vi "OdaNaRadost.vi"(11 "NXT/EV3":T1) -> (3 "NXT/EV3 2":T1)   [LabVIEW 2016]
uses:
  <vilib>/NXT/Subs/LVHSConnector.ctl
  <vilib>/NXT/LegoClasses/BrickReference/BrickReference.lvclass
  <vilib>/NXT/Block Support/NXT_OutputPort.ctl
  <vilib>/NXT/Dual Mode Library/Display/drawText_Center.vi
  <vilib>/NXT/Dual Mode Library/Sound/PlayE.vi
  <vilib>/NXT/Dual Mode Library/Sound/PlayF.vi
  <vilib>/NXT/Dual Mode Library/Sound/PlayG.vi
  <vilib>/NXT/Dual Mode Library/Sound/PlayD.vi
  <vilib>/NXT/Dual Mode Library/Sound/PlayC.vi
  <vilib>/NXT/Dual Mode Library/Waits/Wait_Num.vi
  <vilib>/NXT/NXTIO Xnodes/NXTIONodeSubVIs/NXTMoveMotors.vi
  <vilib>/NXT/NXTIO Xnodes/NXTIONodeSubVIs/NXTStopMotors.vi
  <vilib>/NXT/NXTIO Xnodes/AddressXNode/NXTIOAddress.xnode
  <vilib>/NXT/NXTIO Xnodes/NXTIOXNode/NXTIO.xnode
panel:
  in  "Poèet opakování":i32
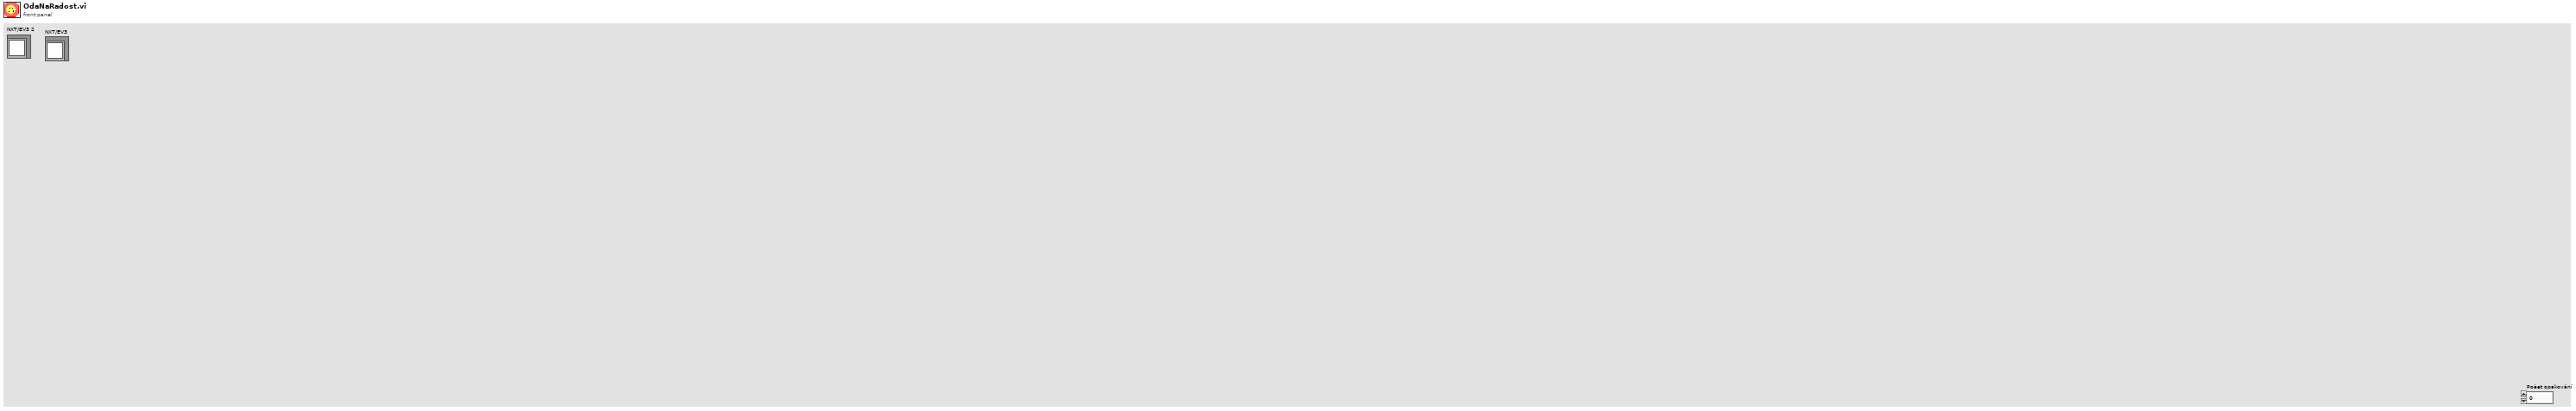
[diagram p1: front panel]
types:
  T1 = typedef "LVHSConnector.ctl" = refnum<class "BrickReference.lvclass">
  T2 = typedef "NXT_OutputPort.ctl" = u8
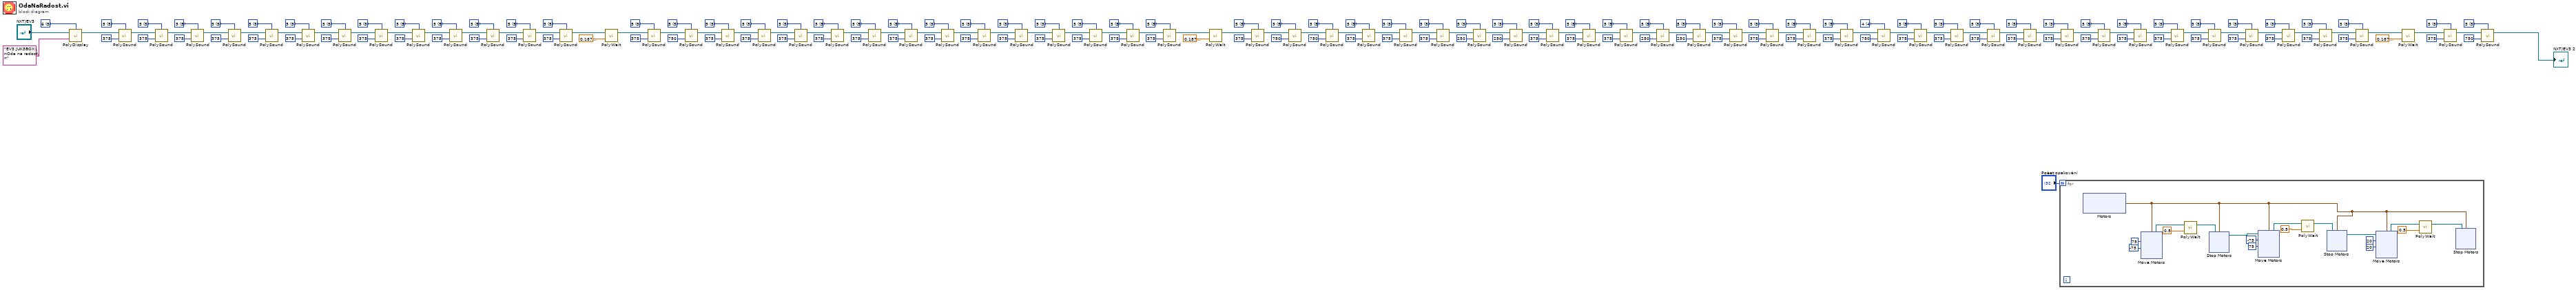
[diagram p0: block diagram]
diagram:
  w47 = u16 5 items=["3"=3, "4"=4, "5"=5, "6"=6, "7"=7] ("Octave")
  w50 = u16 5 items=["3"=3, "4"=4, "5"=5, "6"=6, "7"=7] ("Octave")
  w41 = u16 5 items=["3"=3, "4"=4, "5"=5, "6"=6, "7"=7] ("Octave")
  w36 = u16 5 items=["3"=3, "4"=4, "5"=5, "6"=6, "7"=7] ("Octave")
  w33 = u16 5 items=["3"=3, "4"=4, "5"=5, "6"=6, "7"=7] ("Octave")
  w32 = u16 5 items=["3"=3, "4"=4, "5"=5, "6"=6, "7"=7] ("Octave")
  w29 = u16 5 items=["3"=3, "4"=4, "5"=5, "6"=6, "7"=7] ("Octave")
  w20 = u16 5 items=["3"=3, "4"=4, "5"=5, "6"=6, "7"=7] ("Octave")
  w23 = u16 5 items=["3"=3, "4"=4, "5"=5, "6"=6, "7"=7] ("Octave")
  w24 = u16 5 items=["3"=3, "4"=4, "5"=5, "6"=6, "7"=7] ("Octave")
  w27 = u16 5 items=["3"=3, "4"=4, "5"=5, "6"=6, "7"=7] ("Octave")
  w13 = u16 5 items=["3"=3, "4"=4, "5"=5, "6"=6, "7"=7] ("Octave")
  w10 = u16 5 items=["3"=3, "4"=4, "5"=5, "6"=6, "7"=7] ("Octave")
  w9 = u16 5 items=["3"=3, "4"=4, "5"=5, "6"=6, "7"=7] ("Octave")
  w6 = u16 5 items=["3"=3, "4"=4, "5"=5, "6"=6, "7"=7] ("Octave")
  w53 = u16 4 items=["3"=3, "4"=4, "5"=5, "6"=6, "7"=7] ("Octave")
  w60 = u16 5 items=["3"=3, "4"=4, "5"=5, "6"=6, "7"=7] ("Octave")
  w67 = u16 5 items=["3"=3, "4"=4, "5"=5, "6"=6, "7"=7] ("Octave")
  w70 = u16 5 items=["3"=3, "4"=4, "5"=5, "6"=6, "7"=7] ("Octave")
  w71 = u16 5 items=["3"=3, "4"=4, "5"=5, "6"=6, "7"=7] ("Octave")
  w74 = u16 5 items=["3"=3, "4"=4, "5"=5, "6"=6, "7"=7] ("Octave")
  w57 = u16 5 items=["3"=3, "4"=4, "5"=5, "6"=6, "7"=7] ("Octave")
  w54 = u16 5 items=["3"=3, "4"=4, "5"=5, "6"=6, "7"=7] ("Octave")
  w91 = u16 5 items=["3"=3, "4"=4, "5"=5, "6"=6, "7"=7] ("Octave")
  w94 = u16 5 items=["3"=3, "4"=4, "5"=5, "6"=6, "7"=7] ("Octave")
  w95 = u16 5 items=["3"=3, "4"=4, "5"=5, "6"=6, "7"=7] ("Octave")
  w98 = u16 5 items=["3"=3, "4"=4, "5"=5, "6"=6, "7"=7] ("Octave")
  w84 = u16 5 items=["3"=3, "4"=4, "5"=5, "6"=6, "7"=7] ("Octave")
  w81 = u16 5 items=["3"=3, "4"=4, "5"=5, "6"=6, "7"=7] ("Octave")
  w80 = u16 5 items=["3"=3, "4"=4, "5"=5, "6"=6, "7"=7] ("Octave")
  w77 = u16 5 items=["3"=3, "4"=4, "5"=5, "6"=6, "7"=7] ("Octave")
  w142 = u16 5 items=["3"=3, "4"=4, "5"=5, "6"=6, "7"=7] ("Octave")
  w145 = u16 5 items=["3"=3, "4"=4, "5"=5, "6"=6, "7"=7] ("Octave")
  w136 = u16 5 items=["3"=3, "4"=4, "5"=5, "6"=6, "7"=7] ("Octave")
  w131 = u16 5 items=["3"=3, "4"=4, "5"=5, "6"=6, "7"=7] ("Octave")
  w128 = u16 5 items=["3"=3, "4"=4, "5"=5, "6"=6, "7"=7] ("Octave")
  w127 = u16 5 items=["3"=3, "4"=4, "5"=5, "6"=6, "7"=7] ("Octave")
  w124 = u16 5 items=["3"=3, "4"=4, "5"=5, "6"=6, "7"=7] ("Octave")
  w115 = u16 5 items=["3"=3, "4"=4, "5"=5, "6"=6, "7"=7] ("Octave")
  w118 = u16 5 items=["3"=3, "4"=4, "5"=5, "6"=6, "7"=7] ("Octave")
  w119 = u16 5 items=["3"=3, "4"=4, "5"=5, "6"=6, "7"=7] ("Octave")
  w122 = u16 5 items=["3"=3, "4"=4, "5"=5, "6"=6, "7"=7] ("Octave")
  w108 = u16 5 items=["3"=3, "4"=4, "5"=5, "6"=6, "7"=7] ("Octave")
  w105 = u16 5 items=["3"=3, "4"=4, "5"=5, "6"=6, "7"=7] ("Octave")
  w104 = u16 5 items=["3"=3, "4"=4, "5"=5, "6"=6, "7"=7] ("Octave")
  w101 = u16 5 items=["3"=3, "4"=4, "5"=5, "6"=6, "7"=7] ("Octave")
  w151 = u16 5 items=["3"=3, "4"=4, "5"=5, "6"=6, "7"=7] ("Octave")
  w148 = u16 5 items=["3"=3, "4"=4, "5"=5, "6"=6, "7"=7] ("Octave")
  w157 = u16 5 items=["3"=3, "4"=4, "5"=5, "6"=6, "7"=7] ("Octave")
  w162 = u16 5 items=["3"=3, "4"=4, "5"=5, "6"=6, "7"=7] ("Octave")
  w165 = u16 5 items=["3"=3, "4"=4, "5"=5, "6"=6, "7"=7] ("Octave")
  w166 = u16 5 items=["3"=3, "4"=4, "5"=5, "6"=6, "7"=7] ("Octave")
  w169 = u16 5 items=["3"=3, "4"=4, "5"=5, "6"=6, "7"=7] ("Octave")
  w178 = u16 5 items=["3"=3, "4"=4, "5"=5, "6"=6, "7"=7] ("Octave")
  w175 = u16 5 items=["3"=3, "4"=4, "5"=5, "6"=6, "7"=7] ("Octave")
  w174 = u16 5 items=["3"=3, "4"=4, "5"=5, "6"=6, "7"=7] ("Octave")
  w171 = u16 5 items=["3"=3, "4"=4, "5"=5, "6"=6, "7"=7] ("Octave")
  w185 = u16 5 items=["3"=3, "4"=4, "5"=5, "6"=6, "7"=7] ("Octave")
  w188 = u16 5 items=["3"=3, "4"=4, "5"=5, "6"=6, "7"=7] ("Octave")
  w189 = u16 5 items=["3"=3, "4"=4, "5"=5, "6"=6, "7"=7] ("Octave")
  w192 = u16 5 items=["3"=3, "4"=4, "5"=5, "6"=6, "7"=7] ("Octave")
  w193 = i16 5 items=["1", "2", "3", "4", "5", "6", "7", "8", "9", "10", "11", "12"] ("Line")
  n1 = call-poly <vilib>:"PolyDisplay.vi"("Text"="EV3 JUK3BOX:\nOda na radost\n", "NXT/EV3"="NXT/EV3", "Line"=w193) -> ("NXT/EV3"=w2:T1)  [unwired: 1 in]
  n2 = call-poly <vilib>:"PolySound.vi"("Duration (500 ms)"=u16 375, "NXT/EV3"=w2, "Octave"=w192) -> ("NXT/EV3"=w184:T1)  [unwired: 1 in]
  n3 = call-poly <vilib>:"PolySound.vi"("Duration (500 ms)"=u16 375, "NXT/EV3"=w184, "Octave"=w189) -> ("NXT/EV3"=w183:T1)  [unwired: 1 in]
  n4 = call-poly <vilib>:"PolySound.vi"("Duration (500 ms)"=u16 375, "NXT/EV3"=w183, "Octave"=w188) -> ("NXT/EV3"=w182:T1)  [unwired: 1 in]
  n5 = call-poly <vilib>:"PolySound.vi"("Duration (500 ms)"=u16 375, "NXT/EV3"=w182, "Octave"=w185) -> ("NXT/EV3"=w170:T1)  [unwired: 1 in]
  n6 = call-poly <vilib>:"PolySound.vi"("Duration (500 ms)"=u16 375, "NXT/EV3"=w170, "Octave"=w171) -> ("NXT/EV3"=w179:T1)  [unwired: 1 in]
  n7 = call-poly <vilib>:"PolySound.vi"("Duration (500 ms)"=u16 375, "NXT/EV3"=w179, "Octave"=w174) -> ("NXT/EV3"=w180:T1)  [unwired: 1 in]
  n8 = call-poly <vilib>:"PolySound.vi"("Duration (500 ms)"=u16 375, "NXT/EV3"=w180, "Octave"=w175) -> ("NXT/EV3"=w181:T1)  [unwired: 1 in]
  n9 = call-poly <vilib>:"PolySound.vi"("Duration (500 ms)"=u16 375, "NXT/EV3"=w181, "Octave"=w178) -> ("NXT/EV3"=w158:T1)  [unwired: 1 in]
  n10 = call-poly <vilib>:"PolySound.vi"("Duration (500 ms)"=u16 375, "NXT/EV3"=w158, "Octave"=w169) -> ("NXT/EV3"=w161:T1)  [unwired: 1 in]
  n11 = call-poly <vilib>:"PolySound.vi"("Duration (500 ms)"=u16 375, "NXT/EV3"=w161, "Octave"=w166) -> ("NXT/EV3"=w160:T1)  [unwired: 1 in]
  n12 = call-poly <vilib>:"PolySound.vi"("Duration (500 ms)"=u16 375, "NXT/EV3"=w160, "Octave"=w165) -> ("NXT/EV3"=w159:T1)  [unwired: 1 in]
  n13 = call-poly <vilib>:"PolySound.vi"("Duration (500 ms)"=u16 375, "NXT/EV3"=w159, "Octave"=w162) -> ("NXT/EV3"=w155:T1)  [unwired: 1 in]
  n14 = call-poly <vilib>:"PolySound.vi"("Duration (500 ms)"=u16 375, "NXT/EV3"=w155, "Octave"=w157) -> ("NXT/EV3"=w154:T1)  [unwired: 1 in]
  n15 = call-poly <vilib>:"PolyWait.vi"("Time (1 sec)"=sgl 0.188, "NXT/EV3"=w154) -> ("NXT/EV3"=w147:T1)  [unwired: 2 in]
  n16 = call-poly <vilib>:"PolySound.vi"("Duration (500 ms)"=u16 375, "NXT/EV3"=w147, "Octave"=w148) -> ("NXT/EV3"=w152:T1)  [unwired: 1 in]
  n17 = call-poly <vilib>:"PolySound.vi"("Duration (500 ms)"=u16 750, "NXT/EV3"=w152, "Octave"=w151) -> ("NXT/EV3"=w100:T1)  [unwired: 1 in]
  n18 = call-poly <vilib>:"PolySound.vi"("Duration (500 ms)"=u16 375, "NXT/EV3"=w100, "Octave"=w101) -> ("NXT/EV3"=w109:T1)  [unwired: 1 in]
  n19 = call-poly <vilib>:"PolySound.vi"("Duration (500 ms)"=u16 375, "NXT/EV3"=w109, "Octave"=w104) -> ("NXT/EV3"=w110:T1)  [unwired: 1 in]
  n20 = call-poly <vilib>:"PolySound.vi"("Duration (500 ms)"=u16 375, "NXT/EV3"=w110, "Octave"=w105) -> ("NXT/EV3"=w111:T1)  [unwired: 1 in]
  n21 = call-poly <vilib>:"PolySound.vi"("Duration (500 ms)"=u16 375, "NXT/EV3"=w111, "Octave"=w108) -> ("NXT/EV3"=w123:T1)  [unwired: 1 in]
  n22 = call-poly <vilib>:"PolySound.vi"("Duration (500 ms)"=u16 375, "NXT/EV3"=w123, "Octave"=w122) -> ("NXT/EV3"=w114:T1)  [unwired: 1 in]
  n23 = call-poly <vilib>:"PolySound.vi"("Duration (500 ms)"=u16 375, "NXT/EV3"=w114, "Octave"=w119) -> ("NXT/EV3"=w113:T1)  [unwired: 1 in]
  n24 = call-poly <vilib>:"PolySound.vi"("Duration (500 ms)"=u16 375, "NXT/EV3"=w113, "Octave"=w118) -> ("NXT/EV3"=w112:T1)  [unwired: 1 in]
  n25 = call-poly <vilib>:"PolySound.vi"("Duration (500 ms)"=u16 375, "NXT/EV3"=w112, "Octave"=w115) -> ("NXT/EV3"=w135:T1)  [unwired: 1 in]
  n26 = call-poly <vilib>:"PolySound.vi"("Duration (500 ms)"=u16 375, "NXT/EV3"=w135, "Octave"=w124) -> ("NXT/EV3"=w132:T1)  [unwired: 1 in]
  n27 = call-poly <vilib>:"PolySound.vi"("Duration (500 ms)"=u16 375, "NXT/EV3"=w132, "Octave"=w127) -> ("NXT/EV3"=w133:T1)  [unwired: 1 in]
  n28 = call-poly <vilib>:"PolySound.vi"("Duration (500 ms)"=u16 375, "NXT/EV3"=w133, "Octave"=w128) -> ("NXT/EV3"=w134:T1)  [unwired: 1 in]
  n29 = call-poly <vilib>:"PolySound.vi"("Duration (500 ms)"=u16 375, "NXT/EV3"=w134, "Octave"=w131) -> ("NXT/EV3"=w138:T1)  [unwired: 1 in]
  n30 = call-poly <vilib>:"PolySound.vi"("Duration (500 ms)"=u16 375, "NXT/EV3"=w138, "Octave"=w136) -> ("NXT/EV3"=w139:T1)  [unwired: 1 in]
  n31 = call-poly <vilib>:"PolyWait.vi"("Time (1 sec)"=sgl 0.188, "NXT/EV3"=w139) -> ("NXT/EV3"=w146:T1)  [unwired: 2 in]
  n32 = call-poly <vilib>:"PolySound.vi"("Duration (500 ms)"=u16 375, "NXT/EV3"=w146, "Octave"=w145) -> ("NXT/EV3"=w141:T1)  [unwired: 1 in]
  n33 = call-poly <vilib>:"PolySound.vi"("Duration (500 ms)"=u16 750, "NXT/EV3"=w141, "Octave"=w142) -> ("NXT/EV3"=w76:T1)  [unwired: 1 in]
  n34 = call-poly <vilib>:"PolySound.vi"("Duration (500 ms)"=u16 750, "NXT/EV3"=w76, "Octave"=w77) -> ("NXT/EV3"=w85:T1)  [unwired: 1 in]
  n35 = call-poly <vilib>:"PolySound.vi"("Duration (500 ms)"=u16 375, "NXT/EV3"=w85, "Octave"=w80) -> ("NXT/EV3"=w86:T1)  [unwired: 1 in]
  n36 = call-poly <vilib>:"PolySound.vi"("Duration (500 ms)"=u16 375, "NXT/EV3"=w86, "Octave"=w81) -> ("NXT/EV3"=w87:T1)  [unwired: 1 in]
  n37 = call-poly <vilib>:"PolySound.vi"("Duration (500 ms)"=u16 375, "NXT/EV3"=w87, "Octave"=w84) -> ("NXT/EV3"=w99:T1)  [unwired: 1 in]
  n38 = call-poly <vilib>:"PolySound.vi"("Duration (500 ms)"=u16 250, "NXT/EV3"=w99, "Octave"=w98) -> ("NXT/EV3"=w90:T1)  [unwired: 1 in]
  n39 = call-poly <vilib>:"PolySound.vi"("Duration (500 ms)"=u16 250, "NXT/EV3"=w90, "Octave"=w95) -> ("NXT/EV3"=w89:T1)  [unwired: 1 in]
  n40 = call-poly <vilib>:"PolySound.vi"("Duration (500 ms)"=u16 375, "NXT/EV3"=w89, "Octave"=w94) -> ("NXT/EV3"=w88:T1)  [unwired: 1 in]
  n41 = call-poly <vilib>:"PolySound.vi"("Duration (500 ms)"=u16 375, "NXT/EV3"=w88, "Octave"=w91) -> ("NXT/EV3"=w52:T1)  [unwired: 1 in]
  n42 = call-poly <vilib>:"PolySound.vi"("Duration (500 ms)"=u16 375, "NXT/EV3"=w52, "Octave"=w54) -> ("NXT/EV3"=w58:T1)  [unwired: 1 in]
  n43 = call-poly <vilib>:"PolySound.vi"("Duration (500 ms)"=u16 250, "NXT/EV3"=w58, "Octave"=w57) -> ("NXT/EV3"=w75:T1)  [unwired: 1 in]
  n44 = call-poly <vilib>:"PolySound.vi"("Duration (500 ms)"=u16 250, "NXT/EV3"=w75, "Octave"=w74) -> ("NXT/EV3"=w66:T1)  [unwired: 1 in]
  n45 = call-poly <vilib>:"PolySound.vi"("Duration (500 ms)"=u16 375, "NXT/EV3"=w66, "Octave"=w71) -> ("NXT/EV3"=w65:T1)  [unwired: 1 in]
  n46 = call-poly <vilib>:"PolySound.vi"("Duration (500 ms)"=u16 375, "NXT/EV3"=w65, "Octave"=w70) -> ("NXT/EV3"=w64:T1)  [unwired: 1 in]
  n47 = call-poly <vilib>:"PolySound.vi"("Duration (500 ms)"=u16 375, "NXT/EV3"=w64, "Octave"=w67) -> ("NXT/EV3"=w59:T1)  [unwired: 1 in]
  n48 = call-poly <vilib>:"PolySound.vi"("Duration (500 ms)"=u16 375, "NXT/EV3"=w59, "Octave"=w60) -> ("NXT/EV3"=w63:T1)  [unwired: 1 in]
  n49 = call-poly <vilib>:"PolySound.vi"("Duration (500 ms)"=u16 750, "NXT/EV3"=w63, "Octave"=w53) -> ("NXT/EV3"=w5:T1)  [unwired: 1 in]
  n50 = call-poly <vilib>:"PolySound.vi"("Duration (500 ms)"=u16 375, "NXT/EV3"=w5, "Octave"=w6) -> ("NXT/EV3"=w14:T1)  [unwired: 1 in]
  n51 = call-poly <vilib>:"PolySound.vi"("Duration (500 ms)"=u16 375, "NXT/EV3"=w14, "Octave"=w9) -> ("NXT/EV3"=w15:T1)  [unwired: 1 in]
  n52 = call-poly <vilib>:"PolySound.vi"("Duration (500 ms)"=u16 375, "NXT/EV3"=w15, "Octave"=w10) -> ("NXT/EV3"=w16:T1)  [unwired: 1 in]
  n53 = call-poly <vilib>:"PolySound.vi"("Duration (500 ms)"=u16 375, "NXT/EV3"=w16, "Octave"=w13) -> ("NXT/EV3"=w28:T1)  [unwired: 1 in]
  n54 = for {
    N: "Poèet opakování" -> [_]
    n55 = xnode "Motors"() -> ("Motor"=w198:cluster{"Port":T2, "Port":T2})
    n56 = xnode "Move Motors"("Power/Speed 2"=i8 -75, "Power/Speed 1"=i8 75, "Motors"=w198) -> ("NXT/EV3"=w212:T1)  [unwired: 1 in]
    n57 = call-poly <vilib>:"PolyWait.vi"("Time (1 sec)"=sgl 0.5, "NXT/EV3"=w212) -> ("NXT/EV3"=w211:T1)  [unwired: 2 in]
    n58 = xnode "Stop Motors"("Motors"=w198, "NXT/EV3"=w211) -> ("NXT/EV3"=w204:T1)
    n59 = xnode "Move Motors"("Power/Speed 2"=i8 75, "Power/Speed 1"=i8 -75, "Motors"=w198, "NXT/EV3"=w204) -> ("NXT/EV3"=w205:T1)
    n60 = call-poly <vilib>:"PolyWait.vi"("Time (1 sec)"=sgl 0.5, "NXT/EV3"=w205) -> ("NXT/EV3"=w206:T1)  [unwired: 2 in]
    n61 = xnode "Stop Motors"("Motors"=w198, "NXT/EV3"=w206) -> ("NXT/EV3"=w199:T1)
    n62 = xnode "Move Motors"("Power/Speed 2"=i8 20, "Power/Speed 1"=i8 20, "Motors"=w198, "NXT/EV3"=w199) -> ("NXT/EV3"=w203:T1)
    n63 = call-poly <vilib>:"PolyWait.vi"("Time (1 sec)"=sgl 0.5, "NXT/EV3"=w203) -> ("NXT/EV3"=w202:T1)  [unwired: 2 in]
    n64 = xnode "Stop Motors"("Motors"=w198, "NXT/EV3"=w202) -> ()  [unwired: 1 out]
  }
  n65 = call-poly <vilib>:"PolySound.vi"("Duration (500 ms)"=u16 375, "NXT/EV3"=w28, "Octave"=w27) -> ("NXT/EV3"=w19:T1)  [unwired: 1 in]
  n66 = call-poly <vilib>:"PolySound.vi"("Duration (500 ms)"=u16 375, "NXT/EV3"=w19, "Octave"=w24) -> ("NXT/EV3"=w18:T1)  [unwired: 1 in]
  n67 = call-poly <vilib>:"PolySound.vi"("Duration (500 ms)"=u16 375, "NXT/EV3"=w18, "Octave"=w23) -> ("NXT/EV3"=w17:T1)  [unwired: 1 in]
  n68 = call-poly <vilib>:"PolySound.vi"("Duration (500 ms)"=u16 375, "NXT/EV3"=w17, "Octave"=w20) -> ("NXT/EV3"=w40:T1)  [unwired: 1 in]
  n69 = call-poly <vilib>:"PolySound.vi"("Duration (500 ms)"=u16 375, "NXT/EV3"=w40, "Octave"=w29) -> ("NXT/EV3"=w37:T1)  [unwired: 1 in]
  n70 = call-poly <vilib>:"PolySound.vi"("Duration (500 ms)"=u16 375, "NXT/EV3"=w37, "Octave"=w32) -> ("NXT/EV3"=w38:T1)  [unwired: 1 in]
  n71 = call-poly <vilib>:"PolySound.vi"("Duration (500 ms)"=u16 375, "NXT/EV3"=w38, "Octave"=w33) -> ("NXT/EV3"=w39:T1)  [unwired: 1 in]
  n72 = call-poly <vilib>:"PolySound.vi"("Duration (500 ms)"=u16 375, "NXT/EV3"=w39, "Octave"=w36) -> ("NXT/EV3"=w43:T1)  [unwired: 1 in]
  n73 = call-poly <vilib>:"PolySound.vi"("Duration (500 ms)"=u16 375, "NXT/EV3"=w43, "Octave"=w41) -> ("NXT/EV3"=w44:T1)  [unwired: 1 in]
  n74 = call-poly <vilib>:"PolyWait.vi"("Time (1 sec)"=sgl 0.188, "NXT/EV3"=w44) -> ("NXT/EV3"=w51:T1)  [unwired: 2 in]
  n75 = call-poly <vilib>:"PolySound.vi"("Duration (500 ms)"=u16 375, "NXT/EV3"=w51, "Octave"=w50) -> ("NXT/EV3"=w46:T1)  [unwired: 1 in]
  n76 = call-poly <vilib>:"PolySound.vi"("Duration (500 ms)"=u16 750, "NXT/EV3"=w46, "Octave"=w47) -> ("NXT/EV3"=→"NXT/EV3 2":T1)  [unwired: 1 in]
